vi "Version_4.9_8_on-chip_valves_for25ulSyringe_withModfied_Plunging.vi"() -> ()   [LabVIEW 2020] (continued)
                                }
                                frame "High Resolution Pumping" {
                                n809 = Subtract(x=w1284, y=w1283) -> (x-y=w1280:dbl)
                                n810 = Absolute Value(x=w1280) -> (abs(x)=w1279:dbl)
                                n811 = Multiply(x=w1279, y=w1282) -> (x*y=w1286:dbl)
                                n812 = Divide(x=w1286, y=24000.0) -> (x/y=w1281:dbl)
                                }
                                }
                                n813 = local write "Volume being Injected \nin this process"(w1265) -> ()
                                }
                                frame #1 {
                                n814 = local read "Buffer-C Volume \nto be Pumped for\nColumn \nnon-interference"() -> (w1290:dbl)
                                n815 = local read "Volume being Injected \nin this process"() -> (w1291:dbl)
                                n816 = local read "Stopper that ends \nthe main loops"() -> (w1289:bool)
                                n817 = call "LSPOneStatus (SubVI).vi"("VISA Refnum in"=w1294) -> ("read buffer"=w1296:string)  [unwired: 10 in]
                                n818 = call <vilib>:"Trim Whitespace.vi"("string"=w1296) -> ("trimmed string"=w1295:string)  [unwired: 1 in]
                                n819 = Equal?(x=w1295, y="/0`\u0003") -> (x = y?=w1293:bool)
                                n820 = Greater Or Equal?(x=w1291, y=w1290) -> (x >= y?=w1288:bool)
                                n821 = Or(x=w1289, y=w1288) -> (x .or. y?=w1287:bool)
                                n822 = Or(x=w1293, y=w1287) -> (x .or. y?=w1292:bool)
                                }
                                }
                                n823 = Wait (ms)(milliseconds to wait=u32 100) -> ()  [unwired: 1 out]
                                n824 = local read "Stopper that ends \nthe main loops"() -> (w1257:bool)
                                n825 = case shown="True" w1257 {
                                frame False {
                                }
                                frame True {
                                n826 = local read "VISA Refnum in\nfor Pump"() -> (w1264:refnum<visa-resource-name>)
                                n827 = call "HardStopCurrentProcess (SubVI).vi"("VISA Refnum in"=w1264) -> ()  [unwired: 11 in]
                                }
                                }
                                }
                              }
                              frame #7 {
                                # "Keeps the AMF valve after column-1 closed and valve after column-2 open"
                                n828 = local read "VISA Refnum in\nfor Valve"() -> (w1302:refnum<visa-resource-name>)
                                n829 = local read "External Valve \nCLOSED"() -> (w1301:string)
                                n830 = local write "Valve V4 Open"(TRUE ("Valve V4 Open")) -> ()
                                n831 = local write "Valve V1 Open"(FALSE ("Valve V1 Open")) -> ()
                                n832 = local write "Valve V2 Open"(FALSE ("Valve V2 Open")) -> ()
                                n833 = local write "Valve V3 Open"(FALSE ("Valve V3 Open")) -> ()
                                n834 = call "PortChanger_Valve (SubVI).vi"("Port Number"=w1301, "VISA Refnum in"=w1302) -> ()  [unwired: 10 in]
                                n835 = local write "Valve V7 Open"(TRUE ("Valve V7 Open")) -> ()
                                n836 = local write "Valve V5 Open"(TRUE ("Valve V5 Open")) -> ()
                                n837 = local write "Valve V6 Open"(TRUE ("Valve V6 Open")) -> ()
                              }
                              frame #8 {
                                n838 = local read "Buffer-C1 Pumping\nResolution \nfor Equilibration \nof Column-2"() -> (w1308:T2)
                                n839 = local read "VISA Refnum in\nfor Pump"() -> (w1310:refnum<visa-resource-name>)
                                n840 = local read "Initial Plunger Position"() -> (w1309:dbl)
                                n841 = local read "Volume of Syringe"() -> (w1307:dbl)
                                n842 = while {
                                tunnel: w1309 -> [w1317]
                                tunnel: w1310 -> [w1316]
                                tunnel: w1308 -> [w1315]
                                tunnel: w1307 -> [w1314]
                                stop <- w1312 stop-if-true
                                n843 = stacked-sequence {
                                tunnel: w1317 -> [w1324 _]
                                tunnel: w1316 -> [w1323 w1344]
                                tunnel: w1315 -> [w1322 _]
                                tunnel: w1314 -> [w1321 _]
                                tunnel: [_ w1342] -> w1312
                                frame #0 {
                                n844 = call "AbsolutePlungerPosition (SubVI).vi"("VISA Refnum in"=w1323) -> ("Plunger Position"=w1320:i32)  [unwired: 10 in]
                                n845 = case shown="\"Standard Pumping\", Default" w1322 {
                                tunnel: w1324 -> [w1329 w1338]
                                tunnel: w1320 -> [w1330 w1337]
                                tunnel: [w1328 w1335] -> w1319
                                tunnel: w1321 -> [w1327 w1336]
                                frame "Standard Pumping", Default {
                                n846 = Subtract(x=w1329, y=w1330) -> (x-y=w1326:dbl)
                                n847 = Absolute Value(x=w1326) -> (abs(x)=w1325:dbl)
                                n848 = Multiply(x=w1325, y=w1327) -> (x*y=w1332:dbl)
                                n849 = Divide(x=w1332, y=3000.0) -> (x/y=w1328:dbl)
                                }
                                frame "High Resolution Pumping" {
                                n850 = Subtract(x=w1338, y=w1337) -> (x-y=w1334:dbl)
                                n851 = Absolute Value(x=w1334) -> (abs(x)=w1333:dbl)
                                n852 = Multiply(x=w1333, y=w1336) -> (x*y=w1340:dbl)
                                n853 = Divide(x=w1340, y=24000.0) -> (x/y=w1335:dbl)
                                }
                                }
                                n854 = local write "Volume being Injected \nin this process"(w1319) -> ()
                                }
                                frame #1 {
                                n855 = local read "Stopper that ends \nthe main loops"() -> (w1341:bool)
                                n856 = call "LSPOneStatus (SubVI).vi"("VISA Refnum in"=w1344) -> ("read buffer"=w1346:string)  [unwired: 10 in]
                                n857 = call <vilib>:"Trim Whitespace.vi"("string"=w1346) -> ("trimmed string"=w1345:string)  [unwired: 1 in]
                                n858 = Equal?(x=w1345, y="/0`\u0003") -> (x = y?=w1343:bool)
                                n859 = Or(x=w1343, y=w1341) -> (x .or. y?=w1342:bool)
                                }
                                }
                                n860 = Wait (ms)(milliseconds to wait=u32 100) -> ()  [unwired: 1 out]
                                n861 = local read "Stopper that ends \nthe main loops"() -> (w1311:bool)
                                n862 = case shown="True" w1311 {
                                frame False {
                                }
                                frame True {
                                n863 = local read "VISA Refnum in\nfor Pump"() -> (w1318:refnum<visa-resource-name>)
                                n864 = call "HardStopCurrentProcess (SubVI).vi"("VISA Refnum in"=w1318) -> ()  [unwired: 11 in]
                                }
                                }
                                }
                              }
                              frame #9 {
                                n865 = local write "Pause Data Collection"(TRUE ("Pause Data Collection")) -> ()
                                n866 = Wait (ms)(milliseconds to wait=u32 500) -> ()  [unwired: 1 out]
                              }
                              frame #10 {
                                n867 = local write "Volume being Injected \nin this process"(0.0 ("Volume being Injected \nin this process")) -> ()
                                n868 = local write "Start the Process"(FALSE ("Start the Process")) -> ()
                              }
                            }
                          }
                          frame #10 {
                            # "Clean the tubing with Sample"
                            n869 = local read "N-S"() -> (w1352:i32)
                            n870 = for {
                              N: w1352 -> [_]
                              n871 = stacked-sequence {
                                frame #0 {
                                n872 = local read "VISA Refnum in\nfor Pump"() -> (w1355:refnum<visa-resource-name>)
                                n873 = local read "Port for \nSample"() -> (w1354:string)
                                n874 = call "PortChanger (SubVI).vi"("Port Number"=w1354, "VISA Refnum in"=w1355) -> ()  [unwired: 10 in]
                                }
                                frame #1 {
                                n875 = local read "VISA Refnum in\nfor Pump"() -> (w1356:refnum<visa-resource-name>)
                                n876 = call "ProcessCompletionWaiter (SubVI).vi"("VISA Refnum in"=w1356) -> ()  [unwired: 11 in]
                                }
                                frame #2 {
                                n877 = local read "VISA Refnum in\nfor Pump"() -> (w1361:refnum<visa-resource-name>)
                                n878 = local read "Sample PickUp \nFlow Rate (ul/min)"() -> (w1358:dbl)
                                n879 = local read "V-S"() -> (w1357:dbl)
                                n880 = local read "Volume of Syringe"() -> (w1359:dbl)
                                n881 = call "RPickUp(SubVI).vi"("Volume to be picked up"=w1357, "Volume of Syringe"=w1359, "Resolution of PickUP"=T2."Standard Pumping", "PickUp Flow Rate (ul/min)"=w1358, "VISA Refnum in"=w1361) -> ()  [unwired: 6 in, 1 out]
                                }
                                frame #3 {
                                n882 = local read "Stopper that ends \nthe main loops"() -> (w1362:bool)
                                n883 = local read "VISA Refnum in\nfor Pump"() -> (w1363:refnum<visa-resource-name>)
                                n884 = case shown="True" w1362 {
                                frame False {
                                }
                                frame True {
                                n885 = local read "VISA Refnum in\nfor Pump"() -> (w1364:refnum<visa-resource-name>)
                                n886 = call "HardStopCurrentProcess (SubVI).vi"("VISA Refnum in"=w1364) -> ()  [unwired: 11 in]
                                }
                                }
                                n887 = call "ProcessCompletionWaiter (SubVI).vi"("VISA Refnum in"=w1363) -> ()  [unwired: 11 in]
                                }
                                frame #4 {
                                n888 = local read "VISA Refnum in\nfor Pump"() -> (w1366:refnum<visa-resource-name>)
                                n889 = call "PortChanger (SubVI).vi"("Port Number"="1", "VISA Refnum in"=w1366) -> ()  [unwired: 10 in]
                                }
                                frame #5 {
                                n890 = local read "Stopper that ends \nthe main loops"() -> (w1367:bool)
                                n891 = local read "VISA Refnum in\nfor Pump"() -> (w1368:refnum<visa-resource-name>)
                                n892 = case shown="True" w1367 {
                                frame False {
                                }
                                frame True {
                                n893 = local read "VISA Refnum in\nfor Pump"() -> (w1369:refnum<visa-resource-name>)
                                n894 = call "HardStopCurrentProcess (SubVI).vi"("VISA Refnum in"=w1369) -> ()  [unwired: 11 in]
                                }
                                }
                                n895 = call "ProcessCompletionWaiter (SubVI).vi"("VISA Refnum in"=w1368) -> ()  [unwired: 11 in]
                                }
                                frame #6 {
                                n896 = local read "VISA Refnum in\nfor Pump"() -> (w1374:refnum<visa-resource-name>)
                                n897 = local read "Volume of Syringe"() -> (w1371:dbl)
                                n898 = call "GoToAbsolutePosition(SubVI).vi"("Absolute Volume Position in Syringe (in ul)"=0.0 ("Volume to be picked up"), "Volume of Syringe"=w1371, "Resolution of Pumping"=T2."Standard Pumping" ("Resolution of PickUP"), "Flow Rate (ul/min)"=150.0 ("PickUp Flow Rate (ul/min)"), "VISA Refnum in"=w1374) -> ()  [unwired: 6 in, 1 out]
                                }
                                frame #7 {
                                n899 = local read "Stopper that ends \nthe main loops"() -> (w1375:bool)
                                n900 = local read "VISA Refnum in\nfor Pump"() -> (w1376:refnum<visa-resource-name>)
                                n901 = case shown="True" w1375 {
                                frame False {
                                }
                                frame True {
                                n902 = local read "VISA Refnum in\nfor Pump"() -> (w1377:refnum<visa-resource-name>)
                                n903 = call "HardStopCurrentProcess (SubVI).vi"("VISA Refnum in"=w1377) -> ()  [unwired: 11 in]
                                }
                                }
                                n904 = call "ProcessCompletionWaiter (SubVI).vi"("VISA Refnum in"=w1376) -> ()  [unwired: 11 in]
                                }
                              }
                              n905 = local write "Pause Data Collection"(TRUE ("Pause Data Collection")) -> ()
                            }
                          }
                        }
                        n906 = local write "Equilibriating \nColumn-1"(TRUE ("Equilibriating \nColumn-1")) -> ()
                      }
                      frame #1 {
                        # "Pump Sample into Column-1"
                        n907 = stacked-sequence {
                          frame #0 {
                            # "Switch to Port-3"
                            # "Port-3 of pump is connected to Sample"
                            n908 = local read "VISA Refnum in\nfor Pump"() -> (w1382:refnum<visa-resource-name>)
                            n909 = local read "Port for \nSample"() -> (w1381:string)
                            n910 = call "PortChanger (SubVI).vi"("Port Number"=w1381, "VISA Refnum in"=w1382) -> ()  [unwired: 10 in]
                          }
                          frame #1 {
                            n911 = local read "VISA Refnum in\nfor Pump"() -> (w1383:refnum<visa-resource-name>)
                            n912 = call "ProcessCompletionWaiter (SubVI).vi"("VISA Refnum in"=w1383) -> ()  [unwired: 11 in]
                          }
                          frame #2 {
                            # "V4 is open"
                            # "V1, V2 and V3 are closed"
                            n913 = local read "VISA Refnum in\nfor Valve"() -> (w1388:refnum<visa-resource-name>)
                            n914 = local read "External Valve \nOPEN"() -> (w1387:string)
                            n915 = local write "Valve V1 Open"(TRUE ("Valve V1 Open")) -> ()
                            n916 = local write "Valve V2 Open"(TRUE ("Valve V2 Open")) -> ()
                            n917 = local write "Valve V3 Open"(FALSE ("Valve V3 Open")) -> ()
                            n918 = local write "Valve V4 Open"(FALSE ("Valve V4 Open")) -> ()
                            n919 = call "PortChanger_Valve (SubVI).vi"("Port Number"=w1387, "VISA Refnum in"=w1388) -> ()  [unwired: 10 in]
                            n920 = local write "Valve V5 Open"(FALSE ("Valve V5 Open")) -> ()
                            n921 = local write "Valve V6 Open"(FALSE ("Valve V6 Open")) -> ()
                            n922 = local write "Valve V7 Open"(FALSE ("Valve V7 Open")) -> ()
                          }
                          frame #3 {
                            n923 = local read "Apparent Volume\nof Syringe"() -> (w1393:dbl)
                            n924 = local read "Sample Volume \nto be Pumped"() -> (w1396:dbl)
                            n925 = Quotient & Remainder(x=w1396, y=w1393) -> (x-y*floor(x/y)=w1394:dbl, floor(x/y)=w1395:dbl)
                            n926 = for {
                              N: w1395 -> [_]
                              n927 = stacked-sequence {
                                frame #0 {
                                n928 = local read "Sample PickUp \nFlow Rate (ul/min)"() -> (w1399:dbl)
                                n929 = local read "Sample Pumping\nResolution"() -> (w1398:T2)
                                n930 = local read "VISA Refnum in\nfor Pump"() -> (w1401:refnum<visa-resource-name>)
                                n931 = local read "Apparent Volume\nof Syringe"() -> (w1397:dbl)
                                n932 = local read "Volume of Syringe"() -> (w1400:dbl)
                                n933 = call "RPickUp(SubVI).vi"("Volume to be picked up"=w1397, "Volume of Syringe"=w1400, "Resolution of PickUP"=w1398, "PickUp Flow Rate (ul/min)"=w1399, "VISA Refnum in"=w1401) -> ()  [unwired: 6 in, 1 out]
                                }
                                frame #1 {
                                n934 = local read "Stopper that ends \nthe main loops"() -> (w1402:bool)
                                n935 = local read "VISA Refnum in\nfor Pump"() -> (w1403:refnum<visa-resource-name>)
                                n936 = case shown="True" w1402 {
                                frame False {
                                }
                                frame True {
                                n937 = local read "VISA Refnum in\nfor Pump"() -> (w1404:refnum<visa-resource-name>)
                                n938 = call "HardStopCurrentProcess (SubVI).vi"("VISA Refnum in"=w1404) -> ()  [unwired: 11 in]
                                }
                                }
                                n939 = call "ProcessCompletionWaiter (SubVI).vi"("VISA Refnum in"=w1403) -> ()  [unwired: 11 in]
                                }
                                frame #2 {
                                # "Reads the initial Plunger Position for computing the volume dispensed"
                                n940 = local read "VISA Refnum in\nfor Pump"() -> (w1406:refnum<visa-resource-name>)
                                n941 = call "AbsolutePlungerPosition (SubVI).vi"("VISA Refnum in"=w1406) -> ("Plunger Position"=w1405:i32)  [unwired: 10 in]
                                n942 = local write "Initial Plunger Position"(w1405) -> ()
                                }
                                frame #3 {
                                # "Switch to Port-2"
                                # "Port-2 of the pump is conncted to column-1 of chip"
                                n943 = local read "VISA Refnum in\nfor Pump"() -> (w1408:refnum<visa-resource-name>)
                                n944 = call "PortChanger (SubVI).vi"("Port Number"="2", "VISA Refnum in"=w1408) -> ()  [unwired: 10 in]
                                }
                                frame #4 {
                                n945 = local read "Stopper that ends \nthe main loops"() -> (w1409:bool)
                                n946 = local read "VISA Refnum in\nfor Pump"() -> (w1410:refnum<visa-resource-name>)
                                n947 = case shown="True" w1409 {
                                frame False {
                                }
                                frame True {
                                n948 = local read "VISA Refnum in\nfor Pump"() -> (w1411:refnum<visa-resource-name>)
                                n949 = call "HardStopCurrentProcess (SubVI).vi"("VISA Refnum in"=w1411) -> ()  [unwired: 11 in]
                                }
                                }
                                n950 = call "ProcessCompletionWaiter (SubVI).vi"("VISA Refnum in"=w1410) -> ()  [unwired: 11 in]
                                }
                                frame #5 {
                                # "Keeps the AMF valve after column-1 open and valve after column-2 closed"
                                n951 = local read "Sample Dispense\nFlow Rate (ul/min)"() -> (w1415:dbl)
                                n952 = local read "Sample Pumping\nResolution"() -> (w1414:T2)
                                n953 = local read "VISA Refnum in\nfor Pump"() -> (w1417:refnum<visa-resource-name>)
                                n954 = local write "Pause Data Collection"(FALSE ("Pause Data Collection")) -> ()
                                n955 = local read "Volume of Syringe"() -> (w1416:dbl)
                                n956 = call "GoToAbsolutePosition(SubVI).vi"("Absolute Volume Position in Syringe (in ul)"=0.0 ("Volume to be Dispensed"), "Volume of Syringe"=w1416, "Resolution of Pumping"=w1414, "Flow Rate (ul/min)"=w1415, "VISA Refnum in"=w1417) -> ()  [unwired: 6 in, 1 out]
                                }
                                frame #6 {
                                n957 = local read "Sample Pumping\nResolution"() -> (w1419:T2)
                                n958 = local read "VISA Refnum in\nfor Pump"() -> (w1421:refnum<visa-resource-name>)
                                n959 = local read "Initial Plunger Position"() -> (w1420:dbl)
                                n960 = local read "Volume of Syringe"() -> (w1418:dbl)
                                n961 = while {
                                tunnel: w1420 -> [w1428]
                                tunnel: w1421 -> [w1427]
                                tunnel: w1419 -> [w1426]
                                tunnel: w1418 -> [w1425]
                                stop <- w1423 stop-if-true
                                n962 = stacked-sequence {
                                tunnel: w1428 -> [w1435 _]
                                tunnel: w1427 -> [w1434 w1455]
                                tunnel: w1426 -> [w1433 _]
                                tunnel: w1425 -> [w1432 _]
                                tunnel: [_ w1453] -> w1423
                                frame #0 {
                                n963 = call "AbsolutePlungerPosition (SubVI).vi"("VISA Refnum in"=w1434) -> ("Plunger Position"=w1431:i32)  [unwired: 10 in]
                                n964 = case shown="\"Standard Pumping\", Default" w1433 {
                                tunnel: w1435 -> [w1440 w1449]
                                tunnel: w1431 -> [w1441 w1448]
                                tunnel: [w1439 w1446] -> w1430
                                tunnel: w1432 -> [w1438 w1447]
                                frame "Standard Pumping", Default {
                                n965 = Subtract(x=w1440, y=w1441) -> (x-y=w1437:dbl)
                                n966 = Absolute Value(x=w1437) -> (abs(x)=w1436:dbl)
                                n967 = Multiply(x=w1436, y=w1438) -> (x*y=w1443:dbl)
                                n968 = Divide(x=w1443, y=3000.0) -> (x/y=w1439:dbl)
                                }
                                frame "High Resolution Pumping" {
                                n969 = Subtract(x=w1449, y=w1448) -> (x-y=w1445:dbl)
                                n970 = Absolute Value(x=w1445) -> (abs(x)=w1444:dbl)
                                n971 = Multiply(x=w1444, y=w1447) -> (x*y=w1451:dbl)
                                n972 = Divide(x=w1451, y=24000.0) -> (x/y=w1446:dbl)
                                }
                                }
                                n973 = local write "Volume being Injected \nin this process"(w1430) -> ()
                                }
                                frame #1 {
                                n974 = call "LSPOneStatus (SubVI).vi"("VISA Refnum in"=w1455) -> ("read buffer"=w1457:string)  [unwired: 10 in]
                                n975 = call <vilib>:"Trim Whitespace.vi"("string"=w1457) -> ("trimmed string"=w1456:string)  [unwired: 1 in]
                                n976 = local read "Stopper that ends \nthe main loops"() -> (w1452:bool)
                                n977 = Equal?(x=w1456, y="/0`\u0003") -> (x = y?=w1454:bool)
                                n978 = Or(x=w1454, y=w1452) -> (x .or. y?=w1453:bool)
                                }
                                }
                                n979 = Wait (ms)(milliseconds to wait=u32 100) -> ()  [unwired: 1 out]
                                n980 = local read "Stopper that ends \nthe main loops"() -> (w1422:bool)
                                n981 = case shown="True" w1422 {
                                frame False {
                                }
                                frame True {
                                n982 = local read "VISA Refnum in\nfor Pump"() -> (w1429:refnum<visa-resource-name>)
                                n983 = call "HardStopCurrentProcess (SubVI).vi"("VISA Refnum in"=w1429) -> ()  [unwired: 11 in]
                                }
                                }
                                }
                                }
                                frame #7 {
                                # "Chnage the pump port back to Sample"
                                n984 = local read "VISA Refnum in\nfor Pump"() -> (w1460:refnum<visa-resource-name>)
                                n985 = local read "Port for \nSample"() -> (w1459:string)
                                n986 = local write "Pause Data Collection"(TRUE ("Pause Data Collection")) -> ()
                                n987 = Wait (ms)(milliseconds to wait=u32 500) -> ()  [unwired: 1 out]
                                n988 = call "PortChanger (SubVI).vi"("Port Number"=w1459, "VISA Refnum in"=w1460) -> ()  [unwired: 10 in]
                                }
                                frame #8 {
                                n989 = local read "VISA Refnum in\nfor Pump"() -> (w1463:refnum<visa-resource-name>)
                                n990 = local write "Volume being Injected \nin this process"(0.0 ("Volume being Injected \nin this process")) -> ()
                                n991 = call "ProcessCompletionWaiter (SubVI).vi"("VISA Refnum in"=w1463) -> ()  [unwired: 11 in]
                                }
                              }
                            }
                            n992 = local write "Reminder of the \nVolume to be \nPumped"(w1394) -> ()
                          }
                          frame #4 {
                            n993 = stacked-sequence {
                              frame #0 {
                                n994 = local read "Sample PickUp \nFlow Rate (ul/min)"() -> (w1467:dbl)
                                n995 = local read "Sample Pumping\nResolution"() -> (w1466:T2)
                                n996 = local read "VISA Refnum in\nfor Pump"() -> (w1469:refnum<visa-resource-name>)
                                n997 = local read "Reminder of the \nVolume to be \nPumped"() -> (w1465:dbl)
                                n998 = local read "Volume of Syringe"() -> (w1468:dbl)
                                n999 = call "RPickUp(SubVI).vi"("Volume to be picked up"=w1465, "Volume of Syringe"=w1468, "Resolution of PickUP"=w1466, "PickUp Flow Rate (ul/min)"=w1467, "VISA Refnum in"=w1469) -> ()  [unwired: 6 in, 1 out]
                              }
                              frame #1 {
                                n1000 = local read "Stopper that ends \nthe main loops"() -> (w1470:bool)
                                n1001 = local read "VISA Refnum in\nfor Pump"() -> (w1471:refnum<visa-resource-name>)
                                n1002 = case shown="True" w1470 {
                                frame False {
                                }
                                frame True {
                                n1003 = local read "VISA Refnum in\nfor Pump"() -> (w1472:refnum<visa-resource-name>)
                                n1004 = call "HardStopCurrentProcess (SubVI).vi"("VISA Refnum in"=w1472) -> ()  [unwired: 11 in]
                                }
                                }
                                n1005 = call "ProcessCompletionWaiter (SubVI).vi"("VISA Refnum in"=w1471) -> ()  [unwired: 11 in]
                              }
                              frame #2 {
                                # "Reads the initial Plunger Position for computing the volume dispensed"
                                n1006 = local read "VISA Refnum in\nfor Pump"() -> (w1474:refnum<visa-resource-name>)
                                n1007 = call "AbsolutePlungerPosition (SubVI).vi"("VISA Refnum in"=w1474) -> ("Plunger Position"=w1473:i32)  [unwired: 10 in]
                                n1008 = local write "Initial Plunger Position"(w1473) -> ()
                              }
                              frame #3 {
                                # "Switch to Port-2"
                                # "Port-2 of the pump is conncted to column-1 of chip"
                                n1009 = local read "VISA Refnum in\nfor Pump"() -> (w1476:refnum<visa-resource-name>)
                                n1010 = call "PortChanger (SubVI).vi"("Port Number"="2", "VISA Refnum in"=w1476) -> ()  [unwired: 10 in]
                              }
                              frame #4 {
                                n1011 = local read "Stopper that ends \nthe main loops"() -> (w1477:bool)
                                n1012 = local read "VISA Refnum in\nfor Pump"() -> (w1478:refnum<visa-resource-name>)
                                n1013 = case shown="True" w1477 {
                                frame False {
                                }
                                frame True {
                                n1014 = local read "VISA Refnum in\nfor Pump"() -> (w1479:refnum<visa-resource-name>)
                                n1015 = call "HardStopCurrentProcess (SubVI).vi"("VISA Refnum in"=w1479) -> ()  [unwired: 11 in]
                                }
                                }
                                n1016 = call "ProcessCompletionWaiter (SubVI).vi"("VISA Refnum in"=w1478) -> ()  [unwired: 11 in]
                              }
                              frame #5 {
                                # "Keeps the AMF valve after column-1 open and valve after column-2 closed"
                                n1017 = local read "Sample Dispense\nFlow Rate (ul/min)"() -> (w1483:dbl)
                                n1018 = local read "Sample Pumping\nResolution"() -> (w1482:T2)
                                n1019 = local read "VISA Refnum in\nfor Pump"() -> (w1485:refnum<visa-resource-name>)
                                n1020 = local write "Pause Data Collection"(FALSE ("Pause Data Collection")) -> ()
                                n1021 = local read "Volume of Syringe"() -> (w1484:dbl)
                                n1022 = call "GoToAbsolutePosition(SubVI).vi"("Absolute Volume Position in Syringe (in ul)"=0.0 ("Volume to be Dispensed"), "Volume of Syringe"=w1484, "Resolution of Pumping"=w1482, "Flow Rate (ul/min)"=w1483, "VISA Refnum in"=w1485) -> ()  [unwired: 6 in, 1 out]
                              }
                              frame #6 {
                                n1023 = local read "Sample Pumping\nResolution"() -> (w1487:T2)
                                n1024 = local read "VISA Refnum in\nfor Pump"() -> (w1489:refnum<visa-resource-name>)
                                n1025 = local read "Initial Plunger Position"() -> (w1488:dbl)
                                n1026 = local read "Volume of Syringe"() -> (w1486:dbl)
                                n1027 = while {
                                tunnel: w1488 -> [w1496]
                                tunnel: w1489 -> [w1495]
                                tunnel: w1487 -> [w1494]
                                tunnel: w1486 -> [w1493]
                                stop <- w1491 stop-if-true
                                n1028 = stacked-sequence {
                                tunnel: w1496 -> [w1503 _]
                                tunnel: w1495 -> [w1502 w1523]
                                tunnel: w1494 -> [w1501 _]
                                tunnel: w1493 -> [w1500 _]
                                tunnel: [_ w1521] -> w1491
                                frame #0 {
                                n1029 = call "AbsolutePlungerPosition (SubVI).vi"("VISA Refnum in"=w1502) -> ("Plunger Position"=w1499:i32)  [unwired: 10 in]
                                n1030 = case shown="\"Standard Pumping\", Default" w1501 {
                                tunnel: w1503 -> [w1508 w1517]
                                tunnel: w1499 -> [w1509 w1516]
                                tunnel: [w1507 w1514] -> w1498
                                tunnel: w1500 -> [w1506 w1515]
                                frame "Standard Pumping", Default {
                                n1031 = Subtract(x=w1508, y=w1509) -> (x-y=w1505:dbl)
                                n1032 = Absolute Value(x=w1505) -> (abs(x)=w1504:dbl)
                                n1033 = Multiply(x=w1504, y=w1506) -> (x*y=w1511:dbl)
                                n1034 = Divide(x=w1511, y=3000.0) -> (x/y=w1507:dbl)
                                }
                                frame "High Resolution Pumping" {
                                n1035 = Subtract(x=w1517, y=w1516) -> (x-y=w1513:dbl)
                                n1036 = Absolute Value(x=w1513) -> (abs(x)=w1512:dbl)
                                n1037 = Multiply(x=w1512, y=w1515) -> (x*y=w1519:dbl)
                                n1038 = Divide(x=w1519, y=24000.0) -> (x/y=w1514:dbl)
                                }
                                }
                                n1039 = local write "Volume being Injected \nin this process"(w1498) -> ()
                                }
                                frame #1 {
                                n1040 = call "LSPOneStatus (SubVI).vi"("VISA Refnum in"=w1523) -> ("read buffer"=w1525:string)  [unwired: 10 in]
                                n1041 = call <vilib>:"Trim Whitespace.vi"("string"=w1525) -> ("trimmed string"=w1524:string)  [unwired: 1 in]
                                n1042 = local read "Stopper that ends \nthe main loops"() -> (w1520:bool)
                                n1043 = Equal?(x=w1524, y="/0`\u0003") -> (x = y?=w1522:bool)
                                n1044 = Or(x=w1522, y=w1520) -> (x .or. y?=w1521:bool)
                                }
                                }
                                n1045 = Wait (ms)(milliseconds to wait=u32 100) -> ()  [unwired: 1 out]
                                n1046 = local read "Stopper that ends \nthe main loops"() -> (w1490:bool)
                                n1047 = case shown="True" w1490 {
                                frame False {
                                }
                                frame True {
                                n1048 = local read "VISA Refnum in\nfor Pump"() -> (w1497:refnum<visa-resource-name>)
                                n1049 = call "HardStopCurrentProcess (SubVI).vi"("VISA Refnum in"=w1497) -> ()  [unwired: 11 in]
                                }
                                }
                                }
                              }
                              frame #7 {
                                n1050 = local write "Pause Data Collection"(TRUE ("Pause Data Collection")) -> ()
                                n1051 = Wait (ms)(milliseconds to wait=u32 500) -> ()  [unwired: 1 out]
                              }
                              frame #8 {
                                n1052 = local write "Volume being Injected \nin this process"(0.0 ("Volume being Injected \nin this process")) -> ()
                              }
                            }
                          }
                        }
                        n1053 = local write "Equilibriating \nColumn-2"(FALSE ("Equilibriating \nColumn-2")) -> ()
                        n1054 = local write "Affinity On"(TRUE ("Affinity On")) -> ()
                        n1055 = local write "Sample pumping \ninto Column-1"(TRUE ("Sample pumping \ninto Column-1")) -> ()
                      }
                      frame #2 {
                        # "Wash Column-1 with Buffer-A2"
                        n1056 = stacked-sequence {
                          frame #0 {
                            # "Switch to Port-4/6"
                            # "Port-4/6 of pump is connected to Buffer-A2"
                            n1057 = local read "VISA Refnum in\nfor Pump"() -> (w1533:refnum<visa-resource-name>)
                            n1058 = local read "Port for \nA2-Wash"() -> (w1532:string)
                            n1059 = call "PortChanger (SubVI).vi"("Port Number"=w1532, "VISA Refnum in"=w1533) -> ()  [unwired: 10 in]
                          }
                          frame #1 {
                            n1060 = local read "VISA Refnum in\nfor Pump"() -> (w1534:refnum<visa-resource-name>)
                            n1061 = call "ProcessCompletionWaiter (SubVI).vi"("VISA Refnum in"=w1534) -> ()  [unwired: 11 in]
                          }
                          frame #2 {
                            n1062 = local read "VISA Refnum in\nfor Valve"() -> (w1538:refnum<visa-resource-name>)
                            n1063 = local read "External Valve \nOPEN"() -> (w1539:string)
                            n1064 = local write "Valve V3 Open"(FALSE ("Valve V3 Open")) -> ()
                            n1065 = local write "Valve V4 Open"(FALSE ("Valve V4 Open")) -> ()
                            n1066 = local write "Valve V1 Open"(TRUE ("Valve V1 Open")) -> ()
                            n1067 = local write "Valve V2 Open"(TRUE ("Valve V2 Open")) -> ()
                            n1068 = call "PortChanger_Valve (SubVI).vi"("Port Number"=w1539, "VISA Refnum in"=w1538) -> ()  [unwired: 10 in]
                            n1069 = local write "Valve V5 Open"(FALSE ("Valve V5 Open")) -> ()
                            n1070 = local write "Valve V6 Open"(FALSE ("Valve V6 Open")) -> ()
                            n1071 = local write "Valve V7 Open"(FALSE ("Valve V7 Open")) -> ()
                          }
                          frame #3 {
                            n1072 = local read "Buffer-A2 Volume \nto be Pumped"() -> (w1547:dbl)
                            n1073 = local read "Apparent Volume\nof Syringe"() -> (w1544:dbl)
                            n1074 = Quotient & Remainder(x=w1547, y=w1544) -> (x-y*floor(x/y)=w1545:dbl, floor(x/y)=w1546:dbl)
                            n1075 = for {
                              N: w1546 -> [_]
                              n1076 = stacked-sequence {
                                frame #0 {
                                n1077 = local read "Buffer-A2 PickUp \nFlow Rate (ul/min)"() -> (w1550:dbl)
                                n1078 = local read "Buffer-A2 Pumping\nResolution"() -> (w1549:T2)
                                n1079 = local read "VISA Refnum in\nfor Pump"() -> (w1552:refnum<visa-resource-name>)
                                n1080 = local read "Apparent Volume\nof Syringe"() -> (w1548:dbl)
                                n1081 = local read "Volume of Syringe"() -> (w1551:dbl)
                                n1082 = call "RPickUp(SubVI).vi"("Volume to be picked up"=w1548, "Volume of Syringe"=w1551, "Resolution of PickUP"=w1549, "PickUp Flow Rate (ul/min)"=w1550, "VISA Refnum in"=w1552) -> ()  [unwired: 6 in, 1 out]
                                }
                                frame #1 {
                                n1083 = local read "Stopper that ends \nthe main loops"() -> (w1553:bool)
                                n1084 = local read "VISA Refnum in\nfor Pump"() -> (w1554:refnum<visa-resource-name>)
                                n1085 = case shown="True" w1553 {
                                frame False {
                                }
                                frame True {
                                n1086 = local read "VISA Refnum in\nfor Pump"() -> (w1555:refnum<visa-resource-name>)
                                n1087 = call "HardStopCurrentProcess (SubVI).vi"("VISA Refnum in"=w1555) -> ()  [unwired: 11 in]
                                }
                                }
                                n1088 = call "ProcessCompletionWaiter (SubVI).vi"("VISA Refnum in"=w1554) -> ()  [unwired: 11 in]
                                }
                                frame #2 {
                                # "Reads the initial Plunger Position for computing the volume dispensed"
                                n1089 = local read "VISA Refnum in\nfor Pump"() -> (w1557:refnum<visa-resource-name>)
                                n1090 = call "AbsolutePlungerPosition (SubVI).vi"("VISA Refnum in"=w1557) -> ("Plunger Position"=w1556:i32)  [unwired: 10 in]
                                n1091 = local write "Initial Plunger Position"(w1556) -> ()
                                }
                                frame #3 {
                                # "Switch to Port-2"
                                # "Port-2 of the pump is conncted to column-1 of chip"
                                n1092 = local read "VISA Refnum in\nfor Pump"() -> (w1559:refnum<visa-resource-name>)
                                n1093 = call "PortChanger (SubVI).vi"("Port Number"="2", "VISA Refnum in"=w1559) -> ()  [unwired: 10 in]
                                }
                                frame #4 {
                                n1094 = local read "Stopper that ends \nthe main loops"() -> (w1560:bool)
                                n1095 = local read "VISA Refnum in\nfor Pump"() -> (w1561:refnum<visa-resource-name>)
                                n1096 = case shown="True" w1560 {
                                frame False {
                                }
                                frame True {
                                n1097 = local read "VISA Refnum in\nfor Pump"() -> (w1562:refnum<visa-resource-name>)
                                n1098 = call "HardStopCurrentProcess (SubVI).vi"("VISA Refnum in"=w1562) -> ()  [unwired: 11 in]
                                }
                                }
                                n1099 = call "ProcessCompletionWaiter (SubVI).vi"("VISA Refnum in"=w1561) -> ()  [unwired: 11 in]
                                }
                                frame #5 {
                                # "Keeps the AMF valve after column-1 open and valve after column-2 closed"
                                n1100 = local read "Buffer-A2 Dispense\nFlow Rate (ul/min)"() -> (w1566:dbl)
                                n1101 = local read "Buffer-A2 Pumping\nResolution"() -> (w1565:T2)
                                n1102 = local read "VISA Refnum in\nfor Pump"() -> (w1568:refnum<visa-resource-name>)
                                n1103 = local write "Pause Data Collection"(FALSE ("Pause Data Collection")) -> ()
                                n1104 = local read "Volume of Syringe"() -> (w1567:dbl)
                                n1105 = call "GoToAbsolutePosition(SubVI).vi"("Absolute Volume Position in Syringe (in ul)"=0.0 ("Volume to be Dispensed"), "Volume of Syringe"=w1567, "Resolution of Pumping"=w1565, "Flow Rate (ul/min)"=w1566, "VISA Refnum in"=w1568) -> ()  [unwired: 6 in, 1 out]
                                }
                                frame #6 {
                                n1106 = local read "Buffer-A2 Pumping\nResolution"() -> (w1570:T2)
                                n1107 = local read "VISA Refnum in\nfor Pump"() -> (w1572:refnum<visa-resource-name>)
                                n1108 = local read "Initial Plunger Position"() -> (w1571:dbl)
                                n1109 = local read "Volume of Syringe"() -> (w1569:dbl)
                                n1110 = while {
                                tunnel: w1571 -> [w1579]
                                tunnel: w1572 -> [w1578]
                                tunnel: w1570 -> [w1577]
                                tunnel: w1569 -> [w1576]
                                stop <- w1574 stop-if-true
                                n1111 = stacked-sequence {
                                tunnel: w1579 -> [w1586 _]
                                tunnel: w1578 -> [w1585 w1606]
                                tunnel: w1577 -> [w1584 _]
                                tunnel: w1576 -> [w1583 _]
                                tunnel: [_ w1604] -> w1574
                                frame #0 {
                                n1112 = call "AbsolutePlungerPosition (SubVI).vi"("VISA Refnum in"=w1585) -> ("Plunger Position"=w1582:i32)  [unwired: 10 in]
                                n1113 = case shown="\"Standard Pumping\", Default" w1584 {
                                tunnel: w1586 -> [w1591 w1600]
                                tunnel: w1582 -> [w1592 w1599]
                                tunnel: [w1590 w1597] -> w1581
                                tunnel: w1583 -> [w1589 w1598]
                                frame "Standard Pumping", Default {
                                n1114 = Subtract(x=w1591, y=w1592) -> (x-y=w1588:dbl)
                                n1115 = Absolute Value(x=w1588) -> (abs(x)=w1587:dbl)
                                n1116 = Multiply(x=w1587, y=w1589) -> (x*y=w1594:dbl)
                                n1117 = Divide(x=w1594, y=3000.0) -> (x/y=w1590:dbl)
                                }
                                frame "High Resolution Pumping" {
                                n1118 = Subtract(x=w1600, y=w1599) -> (x-y=w1596:dbl)
                                n1119 = Absolute Value(x=w1596) -> (abs(x)=w1595:dbl)
                                n1120 = Multiply(x=w1595, y=w1598) -> (x*y=w1602:dbl)
                                n1121 = Divide(x=w1602, y=24000.0) -> (x/y=w1597:dbl)
                                }
                                }
                                n1122 = local write "Volume being Injected \nin this process"(w1581) -> ()
                                }
                                frame #1 {
                                n1123 = call "LSPOneStatus (SubVI).vi"("VISA Refnum in"=w1606) -> ("read buffer"=w1608:string)  [unwired: 10 in]
                                n1124 = call <vilib>:"Trim Whitespace.vi"("string"=w1608) -> ("trimmed string"=w1607:string)  [unwired: 1 in]
                                n1125 = local read "Stopper that ends \nthe main loops"() -> (w1603:bool)
                                n1126 = Equal?(x=w1607, y="/0`\u0003") -> (x = y?=w1605:bool)
                                n1127 = Or(x=w1605, y=w1603) -> (x .or. y?=w1604:bool)
                                }
                                }
                                n1128 = Wait (ms)(milliseconds to wait=u32 100) -> ()  [unwired: 1 out]
                                n1129 = local read "Stopper that ends \nthe main loops"() -> (w1573:bool)
                                n1130 = case shown="True" w1573 {
                                frame False {
                                }
                                frame True {
                                n1131 = local read "VISA Refnum in\nfor Pump"() -> (w1580:refnum<visa-resource-name>)
                                n1132 = call "HardStopCurrentProcess (SubVI).vi"("VISA Refnum in"=w1580) -> ()  [unwired: 11 in]
                                }
                                }
                                }
                                }
                                frame #7 {
                                # "Change the port back to Buffer-A2"
                                n1133 = local read "VISA Refnum in\nfor Pump"() -> (w1611:refnum<visa-resource-name>)
                                n1134 = local read "Port for \nA2-Wash"() -> (w1610:string)
                                n1135 = local write "Pause Data Collection"(TRUE ("Pause Data Collection")) -> ()
                                n1136 = Wait (ms)(milliseconds to wait=u32 500) -> ()  [unwired: 1 out]
                                n1137 = call "PortChanger (SubVI).vi"("Port Number"=w1610, "VISA Refnum in"=w1611) -> ()  [unwired: 10 in]
                                }
                                frame #8 {
                                n1138 = local read "VISA Refnum in\nfor Pump"() -> (w1614:refnum<visa-resource-name>)
                                n1139 = local write "Volume being Injected \nin this process"(0.0 ("Volume being Injected \nin this process")) -> ()
                                n1140 = call "ProcessCompletionWaiter (SubVI).vi"("VISA Refnum in"=w1614) -> ()  [unwired: 11 in]
                                }
                              }
                            }
                            n1141 = local write "Reminder of the \nVolume to be \nPumped"(w1545) -> ()
                          }
                          frame #4 {
                            n1142 = stacked-sequence {
                              frame #0 {
                                n1143 = local read "Buffer-A2 PickUp \nFlow Rate (ul/min)"() -> (w1618:dbl)
                                n1144 = local read "Buffer-A2 Pumping\nResolution"() -> (w1617:T2)
                                n1145 = local read "VISA Refnum in\nfor Pump"() -> (w1620:refnum<visa-resource-name>)
                                n1146 = local read "Reminder of the \nVolume to be \nPumped"() -> (w1616:dbl)
                                n1147 = local read "Volume of Syringe"() -> (w1619:dbl)
                                n1148 = call "RPickUp(SubVI).vi"("Volume to be picked up"=w1616, "Volume of Syringe"=w1619, "Resolution of PickUP"=w1617, "PickUp Flow Rate (ul/min)"=w1618, "VISA Refnum in"=w1620) -> ()  [unwired: 6 in, 1 out]
                              }
                              frame #1 {
                                n1149 = local read "Stopper that ends \nthe main loops"() -> (w1621:bool)
                                n1150 = local read "VISA Refnum in\nfor Pump"() -> (w1622:refnum<visa-resource-name>)
                                n1151 = case shown="True" w1621 {
                                frame False {
                                }
                                frame True {
                                n1152 = local read "VISA Refnum in\nfor Pump"() -> (w1623:refnum<visa-resource-name>)
                                n1153 = call "HardStopCurrentProcess (SubVI).vi"("VISA Refnum in"=w1623) -> ()  [unwired: 11 in]
                                }
                                }
                                n1154 = call "ProcessCompletionWaiter (SubVI).vi"("VISA Refnum in"=w1622) -> ()  [unwired: 11 in]
                              }
                              frame #2 {
                                # "Reads the initial Plunger Position for computing the volume dispensed"
                                n1155 = local read "VISA Refnum in\nfor Pump"() -> (w1625:refnum<visa-resource-name>)
                                n1156 = call "AbsolutePlungerPosition (SubVI).vi"("VISA Refnum in"=w1625) -> ("Plunger Position"=w1624:i32)  [unwired: 10 in]
                                n1157 = local write "Initial Plunger Position"(w1624) -> ()
                              }
                              frame #3 {
                                # "Switch to Port-2"
                                # "Port-2 of the pump is conncted to column-1 of chip"
                                n1158 = local read "VISA Refnum in\nfor Pump"() -> (w1627:refnum<visa-resource-name>)
                                n1159 = call "PortChanger (SubVI).vi"("Port Number"="2", "VISA Refnum in"=w1627) -> ()  [unwired: 10 in]
                              }
                              frame #4 {
                                n1160 = local read "Stopper that ends \nthe main loops"() -> (w1628:bool)
                                n1161 = local read "VISA Refnum in\nfor Pump"() -> (w1629:refnum<visa-resource-name>)
                                n1162 = case shown="True" w1628 {
                                frame False {
                                }
                                frame True {
                                n1163 = local read "VISA Refnum in\nfor Pump"() -> (w1630:refnum<visa-resource-name>)
                                n1164 = call "HardStopCurrentProcess (SubVI).vi"("VISA Refnum in"=w1630) -> ()  [unwired: 11 in]
                                }
                                }
                                n1165 = call "ProcessCompletionWaiter (SubVI).vi"("VISA Refnum in"=w1629) -> ()  [unwired: 11 in]
                              }
                              frame #5 {
                                # "Keeps the AMF valve after column-1 open and valve after column-2 closed"
                                n1166 = local read "Buffer-A2 Dispense\nFlow Rate (ul/min)"() -> (w1634:dbl)
                                n1167 = local read "Buffer-A2 Pumping\nResolution"() -> (w1633:T2)
                                n1168 = local read "VISA Refnum in\nfor Pump"() -> (w1636:refnum<visa-resource-name>)
                                n1169 = local write "Pause Data Collection"(FALSE ("Pause Data Collection")) -> ()
                                n1170 = local read "Volume of Syringe"() -> (w1635:dbl)
                                n1171 = call "GoToAbsolutePosition(SubVI).vi"("Absolute Volume Position in Syringe (in ul)"=0.0 ("Volume to be Dispensed"), "Volume of Syringe"=w1635, "Resolution of Pumping"=w1633, "Flow Rate (ul/min)"=w1634, "VISA Refnum in"=w1636) -> ()  [unwired: 6 in, 1 out]
                              }
                              frame #6 {
                                n1172 = local read "Buffer-A2 Pumping\nResolution"() -> (w1638:T2)
                                n1173 = local read "VISA Refnum in\nfor Pump"() -> (w1640:refnum<visa-resource-name>)
                                n1174 = local read "Initial Plunger Position"() -> (w1639:dbl)
                                n1175 = local read "Volume of Syringe"() -> (w1637:dbl)
                                n1176 = while {
                                tunnel: w1639 -> [w1647]
                                tunnel: w1640 -> [w1646]
                                tunnel: w1638 -> [w1645]
                                tunnel: w1637 -> [w1644]
                                stop <- w1642 stop-if-true
                                n1177 = stacked-sequence {
                                tunnel: w1647 -> [w1654 _]
                                tunnel: w1646 -> [w1653 w1674]
                                tunnel: w1645 -> [w1652 _]
                                tunnel: w1644 -> [w1651 _]
                                tunnel: [_ w1672] -> w1642
                                frame #0 {
                                n1178 = call "AbsolutePlungerPosition (SubVI).vi"("VISA Refnum in"=w1653) -> ("Plunger Position"=w1650:i32)  [unwired: 10 in]
                                n1179 = case shown="\"Standard Pumping\", Default" w1652 {
                                tunnel: w1654 -> [w1659 w1668]
                                tunnel: w1650 -> [w1660 w1667]
                                tunnel: [w1658 w1665] -> w1649
                                tunnel: w1651 -> [w1657 w1666]
                                frame "Standard Pumping", Default {
                                n1180 = Subtract(x=w1659, y=w1660) -> (x-y=w1656:dbl)
                                n1181 = Absolute Value(x=w1656) -> (abs(x)=w1655:dbl)
                                n1182 = Multiply(x=w1655, y=w1657) -> (x*y=w1662:dbl)
                                n1183 = Divide(x=w1662, y=3000.0) -> (x/y=w1658:dbl)
                                }
                                frame "High Resolution Pumping" {
                                n1184 = Subtract(x=w1668, y=w1667) -> (x-y=w1664:dbl)
                                n1185 = Absolute Value(x=w1664) -> (abs(x)=w1663:dbl)
                                n1186 = Multiply(x=w1663, y=w1666) -> (x*y=w1670:dbl)
                                n1187 = Divide(x=w1670, y=24000.0) -> (x/y=w1665:dbl)
                                }
                                }
                                n1188 = local write "Volume being Injected \nin this process"(w1649) -> ()
                                }
                                frame #1 {
                                n1189 = call "LSPOneStatus (SubVI).vi"("VISA Refnum in"=w1674) -> ("read buffer"=w1676:string)  [unwired: 10 in]
                                n1190 = call <vilib>:"Trim Whitespace.vi"("string"=w1676) -> ("trimmed string"=w1675:string)  [unwired: 1 in]
                                n1191 = local read "Stopper that ends \nthe main loops"() -> (w1671:bool)
                                n1192 = Equal?(x=w1675, y="/0`\u0003") -> (x = y?=w1673:bool)
                                n1193 = Or(x=w1673, y=w1671) -> (x .or. y?=w1672:bool)
                                }
                                }
                                n1194 = Wait (ms)(milliseconds to wait=u32 100) -> ()  [unwired: 1 out]
                                n1195 = local read "Stopper that ends \nthe main loops"() -> (w1641:bool)
                                n1196 = case shown="True" w1641 {
                                frame False {
                                }
                                frame True {
                                n1197 = local read "VISA Refnum in\nfor Pump"() -> (w1648:refnum<visa-resource-name>)
                                n1198 = call "HardStopCurrentProcess (SubVI).vi"("VISA Refnum in"=w1648) -> ()  [unwired: 11 in]
                                }
                                }
                                }
                              }
                              frame #7 {
                                n1199 = local write "Pause Data Collection"(TRUE ("Pause Data Collection")) -> ()
                                n1200 = Wait (ms)(milliseconds to wait=u32 500) -> ()  [unwired: 1 out]
                              }
                              frame #8 {
                                n1201 = local write "Volume being Injected \nin this process"(0.0 ("Volume being Injected \nin this process")) -> ()
                                n1202 = local write "Start the Process"(FALSE ("Start the Process")) -> ()
                              }
                            }
                          }
                        }
                        n1203 = local write "Sample pumping \ninto Column-1"(FALSE ("Sample pumping \ninto Column-1")) -> ()
                        n1204 = local write "Washing Column-1"(TRUE ("Washing Column-1")) -> ()
                      }
                      frame #3 {
                        # "Connecting Buffer-C with port-5, cleaning the tubing with Buffer-C1, and washing the Column-2 to get rid of spill out from wash steps of column-1"
                        n1205 = stacked-sequence {
                          frame #0 {
                            # "Switch to Port-5"
                            # "Port-5 of pump is connected to Buffer-C1"
                            n1206 = local read "VISA Refnum in\nfor Pump"() -> (w1685:refnum<visa-resource-name>)
                            n1207 = local read "Port for \nC1-Equilibriation"() -> (w1684:string)
                            n1208 = call "PortChanger (SubVI).vi"("Port Number"=w1684, "VISA Refnum in"=w1685) -> ()  [unwired: 10 in]
                          }
                          frame #1 {
                            n1209 = local read "VISA Refnum in\nfor Pump"() -> (w1686:refnum<visa-resource-name>)
                            n1210 = call "ProcessCompletionWaiter (SubVI).vi"("VISA Refnum in"=w1686) -> ()  [unwired: 11 in]
                          }
                          frame #2 {
                            # "Wash the inside of the pump valve"
                            n1211 = local read "n"() -> (w1687:i32)
                            n1212 = for {
                              N: w1687 -> [_]
                              n1213 = stacked-sequence {
                                frame #0 {
                                n1214 = local read "Buffer-A2 Pumping\nResolution"() -> (w1690:T2)
                                n1215 = local read "VISA Refnum in\nfor Pump"() -> (w1692:refnum<visa-resource-name>)
                                n1216 = local read "V-S"() -> (w1688:dbl)
                                n1217 = local read "Volume of Syringe"() -> (w1691:dbl)
                                n1218 = call "RPickUp(SubVI).vi"("Volume to be picked up"=w1688, "Volume of Syringe"=w1691, "Resolution of PickUP"=w1690, "PickUp Flow Rate (ul/min)"=150.0, "VISA Refnum in"=w1692) -> ()  [unwired: 6 in, 1 out]
                                }
                                frame #1 {
                                n1219 = local read "Stopper that ends \nthe main loops"() -> (w1693:bool)
                                n1220 = local read "VISA Refnum in\nfor Pump"() -> (w1694:refnum<visa-resource-name>)
                                n1221 = case shown="True" w1693 {
                                frame False {
                                }
                                frame True {
                                n1222 = local read "VISA Refnum in\nfor Pump"() -> (w1695:refnum<visa-resource-name>)
                                n1223 = call "HardStopCurrentProcess (SubVI).vi"("VISA Refnum in"=w1695) -> ()  [unwired: 11 in]
                                }
                                }
                                n1224 = call "ProcessCompletionWaiter (SubVI).vi"("VISA Refnum in"=w1694) -> ()  [unwired: 11 in]
                                }
                                frame #2 {
                                # "Switch to Port-1"
                                # "Port-1 of the pump is conncted to waste"
                                n1225 = local read "VISA Refnum in\nfor Pump"() -> (w1697:refnum<visa-resource-name>)
                                n1226 = call "PortChanger (SubVI).vi"("Port Number"="1", "VISA Refnum in"=w1697) -> ()  [unwired: 10 in]
                                }
                                frame #3 {
                                n1227 = local read "Stopper that ends \nthe main loops"() -> (w1698:bool)
                                n1228 = local read "VISA Refnum in\nfor Pump"() -> (w1699:refnum<visa-resource-name>)
                                n1229 = case shown="True" w1698 {
                                frame False {
                                }
                                frame True {
                                n1230 = local read "VISA Refnum in\nfor Pump"() -> (w1700:refnum<visa-resource-name>)
                                n1231 = call "HardStopCurrentProcess (SubVI).vi"("VISA Refnum in"=w1700) -> ()  [unwired: 11 in]
                                }
                                }
                                n1232 = call "ProcessCompletionWaiter (SubVI).vi"("VISA Refnum in"=w1699) -> ()  [unwired: 11 in]
                                }
                                frame #4 {
                                n1233 = local read "Buffer-A2 Pumping\nResolution"() -> (w1703:T2)
                                n1234 = local read "VISA Refnum in\nfor Pump"() -> (w1705:refnum<visa-resource-name>)
                                n1235 = local read "Volume of Syringe"() -> (w1704:dbl)
                                n1236 = call "GoToAbsolutePosition(SubVI).vi"("Absolute Volume Position in Syringe (in ul)"=0.0 ("Volume to be Dispensed"), "Volume of Syringe"=w1704, "Resolution of Pumping"=w1703, "Flow Rate (ul/min)"=150.0, "VISA Refnum in"=w1705) -> ()  [unwired: 6 in, 1 out]
                                }
                                frame #5 {
                                n1237 = local read "VISA Refnum in\nfor Pump"() -> (w1706:refnum<visa-resource-name>)
                                n1238 = call "ProcessCompletionWaiter (SubVI).vi"("VISA Refnum in"=w1706) -> ()  [unwired: 11 in]
                                }
                                frame #6 {
                                # "Change the port back to Buffer-C1"
                                n1239 = local read "VISA Refnum in\nfor Pump"() -> (w1708:refnum<visa-resource-name>)
                                n1240 = local read "Port for \nC1-Equilibriation"() -> (w1707:string)
                                n1241 = call "PortChanger (SubVI).vi"("Port Number"=w1707, "VISA Refnum in"=w1708) -> ()  [unwired: 10 in]
                                }
                                frame #7 {
                                n1242 = local read "VISA Refnum in\nfor Pump"() -> (w1709:refnum<visa-resource-name>)
                                n1243 = call "ProcessCompletionWaiter (SubVI).vi"("VISA Refnum in"=w1709) -> ()  [unwired: 11 in]
                                }
                              }
                            }
                          }
                          frame #3 {
                            # "Wash the pathway between column-2 and column-1 on chip"
                            n1244 = local read "n"() -> (w1710:i32)
                            n1245 = for {
                              N: w1710 -> [_]
                              n1246 = stacked-sequence {
                                frame #0 {
                                n1247 = local read "Buffer-A2 Pumping\nResolution"() -> (w1713:T2)
                                n1248 = local read "VISA Refnum in\nfor Pump"() -> (w1715:refnum<visa-resource-name>)
                                n1249 = local read "V-S"() -> (w1711:dbl)
                                n1250 = local read "Volume of Syringe"() -> (w1714:dbl)
                                n1251 = call "RPickUp(SubVI).vi"("Volume to be picked up"=w1711, "Volume of Syringe"=w1714, "Resolution of PickUP"=w1713, "PickUp Flow Rate (ul/min)"=150.0, "VISA Refnum in"=w1715) -> ()  [unwired: 6 in, 1 out]
                                }
                                frame #1 {
                                n1252 = local read "Stopper that ends \nthe main loops"() -> (w1716:bool)
                                n1253 = local read "VISA Refnum in\nfor Pump"() -> (w1717:refnum<visa-resource-name>)
                                n1254 = case shown="True" w1716 {
                                frame False {
                                }
                                frame True {
                                n1255 = local read "VISA Refnum in\nfor Pump"() -> (w1718:refnum<visa-resource-name>)
                                n1256 = call "HardStopCurrentProcess (SubVI).vi"("VISA Refnum in"=w1718) -> ()  [unwired: 11 in]
                                }
                                }
                                n1257 = call "ProcessCompletionWaiter (SubVI).vi"("VISA Refnum in"=w1717) -> ()  [unwired: 11 in]
                                }
                                frame #2 {
                                # "Switch to Port-10"
                                # "Port-10 of the pump is conncted to column-2"
                                n1258 = local read "VISA Refnum in\nfor Pump"() -> (w1720:refnum<visa-resource-name>)
                                n1259 = call "PortChanger (SubVI).vi"("Port Number"="10", "VISA Refnum in"=w1720) -> ()  [unwired: 10 in]
                                }
                                frame #3 {
                                n1260 = local read "Stopper that ends \nthe main loops"() -> (w1721:bool)
                                n1261 = local read "VISA Refnum in\nfor Pump"() -> (w1722:refnum<visa-resource-name>)
                                n1262 = case shown="True" w1721 {
                                frame False {
                                }
                                frame True {
                                n1263 = local read "VISA Refnum in\nfor Pump"() -> (w1723:refnum<visa-resource-name>)
                                n1264 = call "HardStopCurrentProcess (SubVI).vi"("VISA Refnum in"=w1723) -> ()  [unwired: 11 in]
                                }
                                }
                                n1265 = call "ProcessCompletionWaiter (SubVI).vi"("VISA Refnum in"=w1722) -> ()  [unwired: 11 in]
                                }
                                frame #4 {
                                n1266 = local read "Buffer-A2 Pumping\nResolution"() -> (w1732:T2)
                                n1267 = local read "VISA Refnum in\nfor Pump"() -> (w1734:refnum<visa-resource-name>)
                                n1268 = local read "f"() -> (w1724:dbl)
                                n1269 = local read "Volume of Syringe"() -> (w1733:dbl)
